vi "判断试用期.vi"(8 "error in (no error)":errorcluster caption="错误输入（无错误）", 11 "T":u32) -> (0 "error out":errorcluster caption="错误输出", 3 "试用期内":bool)   [LabVIEW 2014]
panel:
  out "时间标识":timestamp
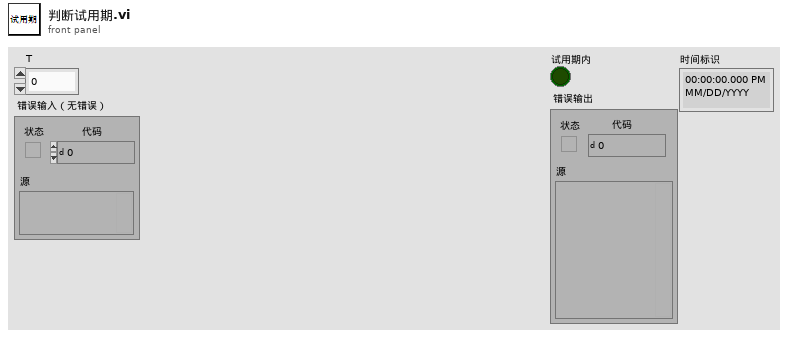
[diagram p1: front panel]
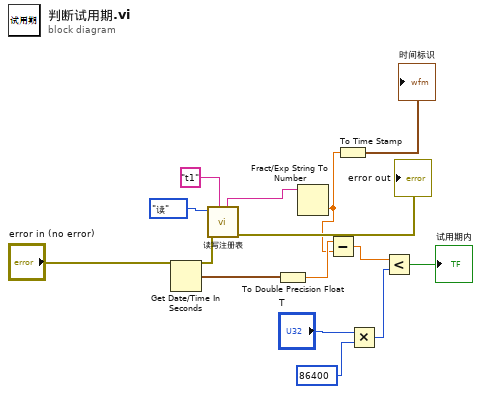
[diagram p0: block diagram]
diagram:
  n1 = Get Date/Time In Seconds() -> (seconds since 1Jan1904=w12:timestamp)
  n2 = call "读写注册表.vi"("键名称"="t1", "error in (no error)"="error in (no error)", "读/写"=enum16{"读", "写"}."读") -> ("error out"=→"error out":errorcluster, "键内容"=w3:string)  [unwired: 7 in]
  n3 = To Double Precision Float(number=w12) -> (double precision float=w11:dbl)
  n4 = Fract/Exp String To Number(string=w3) -> (number=w2:dbl)  [unwired: 3 in, 1 out]
  n5 = Subtract(x=w11, y=w2) -> (x-y=w10:dbl)
  n6 = To Time Stamp(1:w2) -> (0:→"时间标识":timestamp)
  n7 = Multiply(x="T", y=u32 86400) -> (x*y=w7:u32)
  n8 = Less?(x=w10, y=w7) -> (x < y?=→"试用期内":bool)
